vi "Export_JSON.vi"() -> ()   [LabVIEW 2019]
uses:
  MainFGV/Settings/Advanced/AdvancedConfig.ctl
  Processing/results_data.ctl
panel:
  in  "Ensaios":path=path "C:/Users/l01481/Desktop/nada"
  in  "stop":bool
  in  "delete":bool
  in  "ok":bool
  in  "validate":bool
  in  "tab":T1(tab)
  out "inert":waveform(dbl)[](graph) caption="Inertância"
  out "hammerSpec":waveform(dbl)(graph) caption="Martelo - Espectro"
  out "acelTime":waveform(dbl)[](graph) caption="Acelerômetros - Sinal no tempo"
  out "hammerTime":waveform(dbl)(graph) caption="Martelo - Sinal no tempo"
  out "meanInert":picture
  # "Análise modal\n\nAquisição\n\nLink do repositório: https://github.com/LeonardoSirino/ModalAnalysis"
  # "Leonardo Sirino\nSistemas Mecânicos \nT + 55 (41) 3361-6152 | C + 55 (41) 99679-007\nleonardo.sirino@lactec.org.br | www.lactec.org.br"
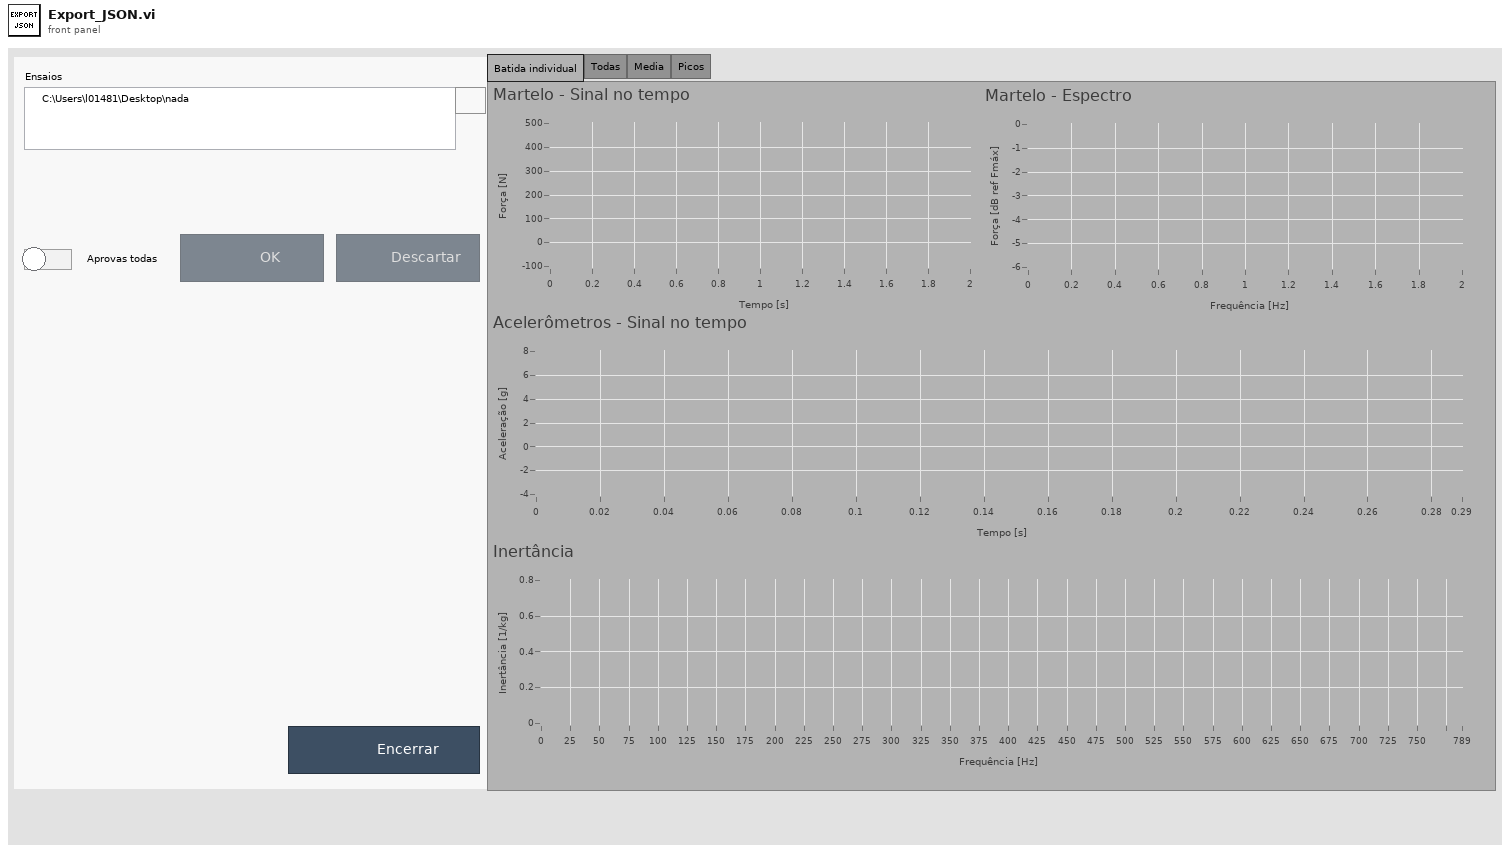
[diagram p1: front panel]
types:
  T1 = enum32{"Batida individual", "Todas", "Media", "Picos"}
  T2 = enum8{"Enabled", "Disabled", "Disabled and Grayed Out"}
  T3 = typedef "results_data.ctl" = cluster{"config":T4, "hammer":waveform(dbl), "acelerometers":waveform(dbl)[], "hammerIndex":i32}
  T4 = typedef "AdvancedConfig.ctl" = cluster{"rate":dbl, "duration":dbl, "thr":dbl, "preTrigger":dbl, "cutoff":dbl, "Filtro":enum16{"Desativado", "Passa banda", "Passa alta", "Passa baixa"}, "highPass":dbl, "lowPass":dbl, "updateTime":dbl}
  T5 = cluster{"seconds since 1Jan1904":timestamp, "data_out":T3}
  T6 = cluster{"seconds since 1Jan1904":timestamp, "data_out":T3}[]
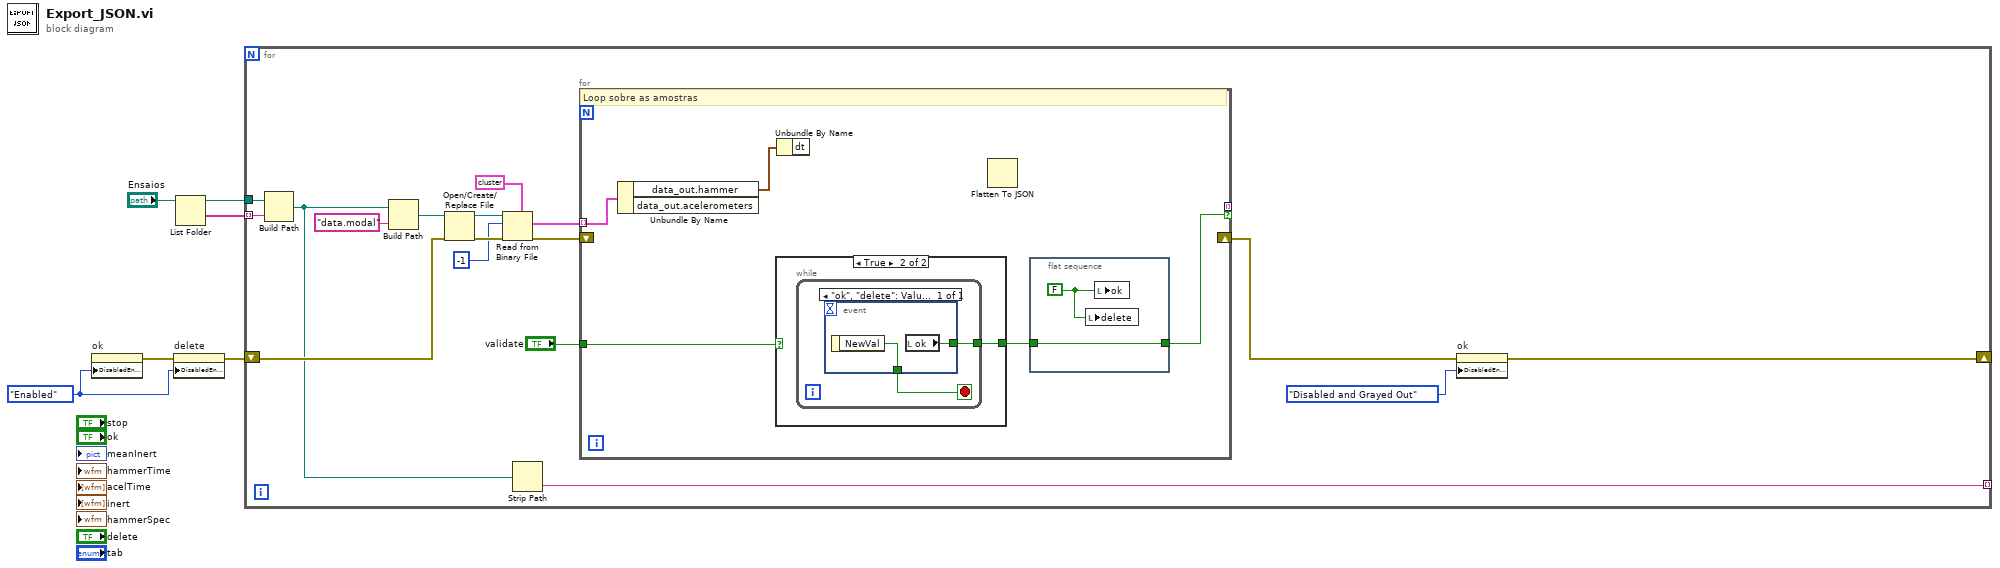
[diagram p0: block diagram]
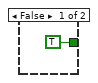
[diagram p2: hidden frame]
diagram:
  w6 = T2."Enabled" ("Disabled")
  n1 = property on="ok" class="Bool (strict)"("DisabledEnum"=w6) -> (error out=w5:errorcluster)  [unwired: 2 in, 1 out]
  n2 = property on="delete" class="Bool (strict)"(error in=w5, "DisabledEnum"=w6) -> (error out=w4:errorcluster)  [unwired: 1 in, 1 out]
  n3 = List Folder(path="Ensaios") -> (path out=w2:path, folder names=w1:string[])  [unwired: 3 in, 2 out]
  n4 = for {
    shift-right: [w7] -> _
    shift-left: w4 -> [w12]
    tunnel: w2 -> [w10]
    tunnel: [w11] -> _ mode=indexing
    tunnel: w1 -> [w9] mode=indexing
    n5 = Build Path(base path=w10, name or relative path=w9) -> (appended path=w8:path)
    n6 = Build Path(base path=w8, name or relative path="data.modal") -> (appended path=w22:path)
    n7 = Open/Create/Replace File(file path (use dialog)=w22, error in=w12) -> (refnum out=w21:refnum<file>, error out=w19:errorcluster)  [unwired: 4 in, 1 out]
    n8 = Read from Binary File(5:T5 {"seconds since 1Jan1904"=timestamp(0 s since 1904-01-01), "data_out"={"config"={"rate"=0.0, "duration"=0.0, "thr"=0.0, "preTrigger"=0.0, "cutoff"=0.0, "Filtro"=enum."Desativado", "highPass"=0.0, "lowPass"=0.0, "updateTime"=0.0}, "hammer"={"t0"=timestamp(0 s since 1904-01-01), "dt"=1.0, "Y"=[]}, "acelerometers"=[], "hammerIndex"=0}} ("output cluster"), 8:w19, 10:-1 ("count (1)"), 11:w21) -> (0:w16:errorcluster, 2:w17:T6)  [unwired: 2 in, 2 out]
    n9 = Strip Path(path=w8) -> (name=w11:string)  [unwired: 1 out]
    n10 = for {
      tunnel: w17 -> [w28] mode=indexing
      shift-right: [_] -> w14
      shift-left: w16 -> [_]
      tunnel: _ -> [_] mode=indexing if=w25
      tunnel: "validate" -> [w24]
      # "Loop sobre as amostras"
      n11 = Unbundle By Name(w28) -> ("data_out.hammer"=w27:waveform(dbl))  [unwired: 1 out]
      n12 = case shown="True" w24 {
        tunnel: [TRUE ("ok") w32] -> w26
        frame False {
        }
        frame True {
          n13 = while {
            tunnel: [w34] -> w32
            stop <- w33 stop-if-true
            n14 = event shown="[0] \"ok\", \"delete\": Value Change" {
              selector: _ -> [_]
              dyn-events: _ -> [_]
              timeout: _ -> [_]
              tunnel: [w35] -> w34
              tunnel: [w36] -> w33
              event "ok", "delete": Value Change {
                n15 = event-data() -> ("NewVal"=w36:bool)  [unwired: 1 in]
                n16 = local read "ok"() -> (w35:bool)
              }
            }
          }
        }
      }
      n17 = Unbundle By Name(w27) -> ()  [unwired: 1 out]
      n18 = Flatten To JSON() -> ()  [unwired: 3 in, 2 out]
      n19 = flat-sequence {
        tunnel: w26 -> [w30]
        tunnel: [w30] -> w25
        frame #0 {
          w29 = FALSE ("ok")
          n20 = local write "delete"(w29) -> ()
          n21 = local write "ok"(w29) -> ()
        }
      }
    }
    n22 = property on="ok" class="Bool (strict)"(error in=w14, "DisabledEnum"=T2."Disabled and Grayed Out" ("Disabled")) -> (error out=w7:errorcluster)  [unwired: 1 in, 1 out]
  }
